vi "Add String.vi"(8 "error in (no error)":errorcluster, 10 "string":string, 11 "Buffer in":refnum<class "Unique String Buffer.lvclass">) -> (0 "error out":errorcluster, 3 "Buffer out":refnum<class "Unique String Buffer.lvclass">)   [LabVIEW 2015, in "SLSC Switch.lvlib" / "Unique String Buffer.lvclass"]
uses:
  Unique String Buffer.lvclass
  Unique String Buffer.lvclass/Unique String Buffer.ctl
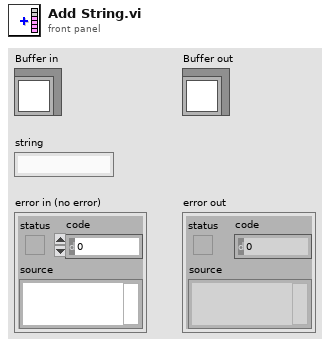
[diagram p1: front panel]
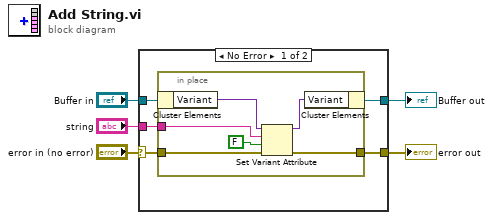
[diagram p0: block diagram]
diagram:
  n1 = case shown="No Error" "error in (no error)" {
    selector: "error in (no error)" -> [w7 w18]
    tunnel: [w6 w18] -> w4
    tunnel: [w8 w17] -> w2
    tunnel: "Buffer in" -> [w10 w17]
    tunnel: "string" -> [w9 _]
    frame No Error {
      n2 = in-place {
        in-place-border: w9 -> [w14]
        in-place-border: w7 -> [w12]
        in-place-border: [w11] -> w6
        n3 = in-place-cluster #1(w10) -> ("Variant"=w16:variant)
        n4 = Set Variant Attribute(Variant=w16, name=w14, value=FALSE, error in=w12) -> (Variant out=w15:variant, error out=w11:errorcluster)  [unwired: 1 out]
        n5 = in-place-cluster #1("Variant"=w15) -> (w8:refnum<class "Unique String Buffer.lvclass">)
      }
    }
    frame Error {
    }
  }
  "error out" <- w4
  "Buffer out" <- w2
